vi "U01_TCP_WHILE.vi"() -> ()   [LabVIEW 2015]
panel:
  out "data out":string
  in  "mode (standard)":T1(ring)
  in  "bytes to read":i32=4
  out "error out":errorcluster
  in  "service name":string
  in  "port":u16
  in  "timeout ms (wait forever: -1)":i32=-1
  in  "error in (no error)":errorcluster
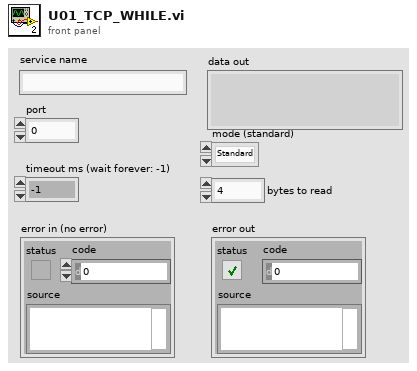
[diagram p1: front panel]
types:
  T1 = enum16{"Standard", "Buffered", "CRLF", "Immediate"}
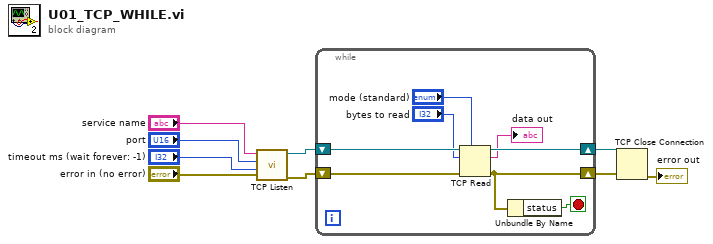
[diagram p0: block diagram]
diagram:
  n1 = call <vilib>:"TCP Listen.vi"("error in (no error)"="error in (no error)", "timeout ms (wait forever: -1)"="timeout ms (wait forever: -1)", "port"="port", "service name"="service name") -> ("error out"=w5:errorcluster, "connection ID"=w4:refnum<k5>)  [unwired: 3 in, 3 out]
  n2 = while {
    shift-right: [w12] -> w3
    shift-left: w5 -> [w17]
    shift-right: [w14] -> w2
    shift-left: w4 -> [w16]
    stop <- w11 stop-if-true
    n3 = TCP Read(connection ID=w16, bytes to read="bytes to read", error in (no error)=w17, 7:"mode (standard)") -> (connection ID out=w14:refnum<k5>, data out=→"data out":string, error out=w12:errorcluster)  [unwired: 1 in]
    n4 = Unbundle By Name(w12) -> ("status"=w11:bool)
  }
  n5 = TCP Close Connection(connection ID=w2, error in (no error)=w3) -> (error out=→"error out":errorcluster)  [unwired: 1 in, 1 out]
